vi "EnFlo_Hub.vi"() -> ()   [LabVIEW 2010]
uses:
  Anemometry Sub Vis/Controls/Launch_controls/Open_Calib.ctl
  Anemometry Sub Vis/Controls/Launch_controls/Open_Meas.ctl
  Anemometry Sub Vis/Controls/Launch_controls/Open_Enter_Temp.ctl
  Anemometry Sub Vis/Controls/Launch_controls/Multi_Run_Prog.ctl
  Anemometry Sub Vis/Controls/Launch_controls/EnFlo_arm.ctl
  Anemometry Sub Vis/Controls/Launch_controls/Fast_FID_Valve.ctl
  Anemometry Sub Vis/Controls/Launch_controls/Disp_Setup.ctl
  Anemometry Sub Vis/Controls/Launch_controls/EnFlo_Tun_Setup.ctl
  Anemometry Sub Vis/Controls/Launch_controls/User_Metadata.ctl
  Anemometry Sub Vis/Controls/Launch_controls/Trav_3D_move.ctl
  Anemometry Sub Vis/Controls/Launch_controls/Trav_Space.ctl
  Anemometry Sub Vis/Controls/Launch_controls/Tunnel_speed.ctl
  Anemometry Sub Vis/Controls/Launch_controls/Client_source_control.ctl
  Anemometry Sub Vis/Controls/Launch_controls/Hydrosonic_Manual.ctl
  Anemometry Sub Vis/Controls/Launch_controls/Preference_Panel.ctl
  Anemometry Sub Vis/Controls/Launch_controls/Hot_wire_Calculator.ctl
  Anemometry Sub Vis/Controls/Launch_controls/RW_X_Parker_Config.ctl
  Anemometry Sub Vis/Controls/Launch_controls/LDA_Alignment.ctl
  Anemometry Sub Vis/Controls/Launch_controls/Named_Serial_Comms.ctl
  Anemometry Sub Vis/Controls/Launch_controls/BSA_data_rates.ctl
  Anemometry Sub Vis/Controls/Launch_controls/Recompile_Code.ctl
  Anemometry Sub Vis/Controls/Launch_controls/Serial_Setup.ctl
  Anemometry Sub Vis/Controls/Launch_controls/Post_Process_icon.ctl
  Anemometry Sub Vis/Controls/Launch_controls/Edit_Ascii_file.ctl
  Anemometry Sub Vis/Controls/Launch_controls/Edit_Raw_DF.ctl
  Anemometry Sub Vis/Controls/Launch_controls/Results_file_plotter.ctl
  Anemometry Sub Vis/Controls/Launch_controls/Serial_Port_Names.ctl
  Anemometry Sub Vis/Controls/Launch_controls/Enter_LDA_Setup.ctl
  Anemometry Sub Vis/Controls/Launch_controls/Paul.ctl
  Anemometry Sub Vis/Controls/Launch_controls/Tom.ctl
  Anemometry Sub Vis/Controls/Launch_controls/Scani_Valve.ctl
  Anemometry Sub Vis/Controls/Launch_controls/Edit_sever_Channel.ctl
  Anemometry Sub Vis/Controls/Launch_controls/Day_file_plotter.ctl
  Anemometry Sub Vis/Controls/Launch_controls/Plot_Sever_Data.ctl
  Anemometry Sub Vis/Controls/Launch_controls/Adam_Table.ctl
  Anemometry Sub Vis/Controls/Launch_controls/Active_Channel_Control.ctl
  Anemometry Sub Vis/Controls/Post_Process.ctl
  Anemometry Sub Vis/Controls/Setup.ctl
  Anemometry Sub Vis/Controls/Preference_Mode.ctl
  Anemometry Sub Vis/Controls/User_Specific_mode.ctl
  Anemometry Sub Vis/Gen Trav/Trav_mode.ctl
  Anemometry Sub Vis/Calibration/Calib_mode.ctl
  Anemometry Sub Vis/Controls/App_Global.ctl
  Anemometry Sub Vis/Globals/Dynamic_call_global.ph.vi
  Anemometry Sub Vis/Globals/Preference_global.vi
  Anemometry Sub Vis/Globals/Constants_global.vi
  Anemometry Sub Vis/Globals/Meas_global.vi
  <vilib>/Platform/browser.llb/Open URL in Default Browser (string).vi
  Anemometry Sub Vis/Globals/Trav_pos_global.vi
  Anemometry Sub Vis/Acquisition/PWA/PWAtasksGLOBAL.vi
  Anemometry Sub Vis/Globals/Qnet_Globals.vi
  Anemometry Sub Vis/Utilities/Email_transfer_global.vi
panel:
  out "List of ADAM channels to view":string[](array[string])
  out "List of ADAM control channels":string[](array[string])
  out "Analogue Dev Name":string="Dev2"
  out "Numeric":i32
  out "Rig Name":string="EnFlo Tunnel"
  out "Meas setups folder":path=path "/System Folder/Preferences/LabVIEW (EnFlo specific)/Meas Setups"
  out "Dummy Measurement":bool
  out "Ready to take data?":T1
  out "Local Site Root":path=path "/Lacie_20/paulhayden/Qnet/qnet"
  in  "stop":bool
  in  "Tab Control":T2(tab)
  in  "Tunnel Speed Control":T3
  in  "Traverse Space":T4
  in  "Trav 3D Move":T5 caption="3D Traverse Move"
  in  "User Metadata":T6
  in  "Multi Run Prog":T7
  in  "Enter Temp_Press":T8
  in  "Measurement Prog":T9 caption="Measurement"
  in  "Calibration Prog":T10 caption="Calibration"
  in  "Scani Valve":T11
  in  "LDA Alignment":T12
  in  "Hydrosonic Control":T13
  in  "Fast FID Valve":T14
  in  "Source Control":T15
  in  "Gas Release Setup":T16
  in  "EnFlo Tunnel Setup":T17
  in  "Heater Setup":bool caption="Inlet heater File"
  in  "EnFlo Arm":T18
  in  "Rig_Control":cluster{"Ch Name":string, "Boolean":bool}[](array[cluster])
  in  "ADAM Channels Control":T19 caption="Change Active Channels"
  in  "ADAM Scan Table":T20 caption="Run ADAM Scan Table"
  in  "Edit Server Channel":T21
  in  "Plot Server Channels":T22 caption="Plot Server Data"
  in  "Day Files Plotter":T23 caption="Plot Data From File"
  out "Current Values":cluster{"Ch Name":string, "Numeric":dbl}[](array[cluster])
  in  "Results File Plotter":T24
  in  "Edit Raw Data Files":T25
  in  "Edit ASCII File":T26
  in  "Post Process Raw Data":T27
  in  "LDA Setup":T28
  in  "Port Names":T29
  in  "Serial Setup":T30
  in  "Software Update":T31
  in  "LDA Data Rate":T32
  in  "Named Serial Comms":T33
  in  "RW Trav Setup":T34
  in  "Hot Wire Calc":T35
  in  "Preference Panel":T36
  in  "Tom Lawton t.lawton@surrey.ac.uk":T37 caption="For hardware support"
  in  "Paul Hayden p.hayden@surrey.ac.uk":T38 caption="For software support"
  in  "Online Manual":bool
  out "VI Name":string
  out "Iterations":i32
  # "Or give us a call on Tel: 01483 689545"
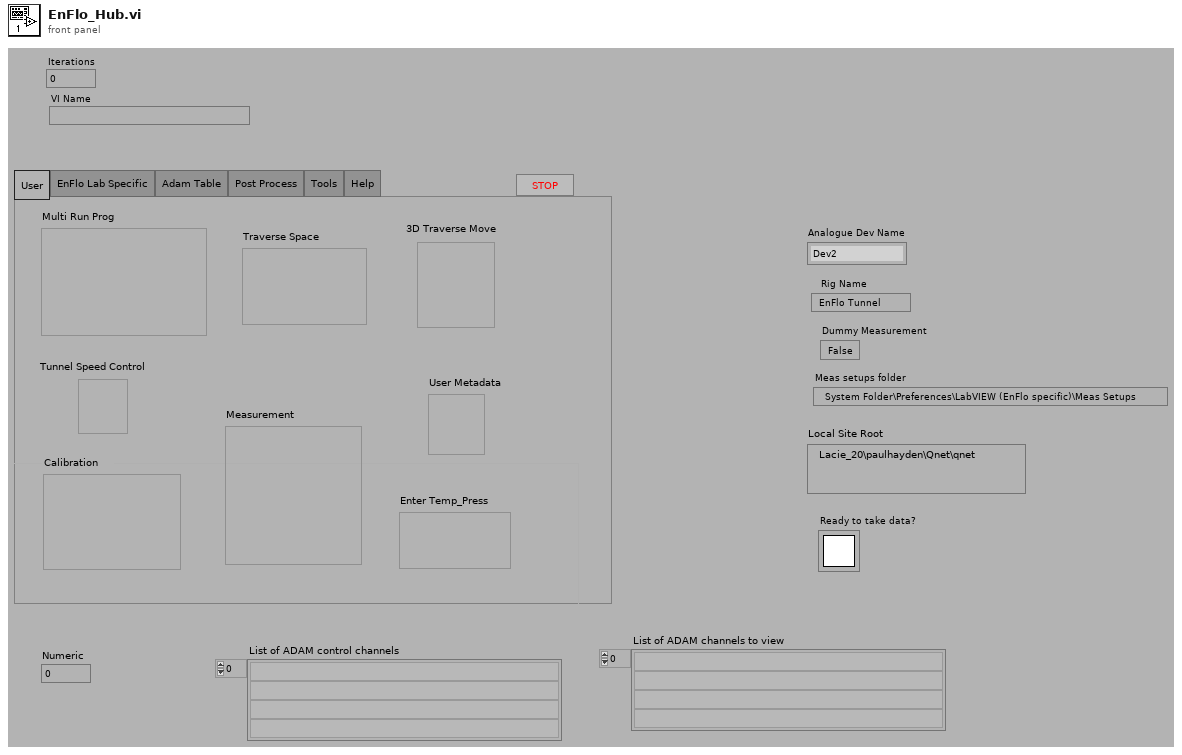
[diagram p1: front panel]
types:
  T1 = typedef "Rendezvous RefNum" = refnum<k1>
  T2 = enum32{"User", "EnFlo Lab Specific", "Adam Table", "Post Process", "Tools", "Help"}
  T3 = typedef "Tunnel_speed.ctl" = bool
  T4 = typedef "Trav_Space.ctl" = bool
  T5 = typedef "Trav_3D_move.ctl" = bool
  T6 = typedef "User_Metadata.ctl" = bool
  T7 = typedef "Multi_Run_Prog.ctl" = bool
  T8 = typedef "Open_Enter_Temp.ctl" = bool
  T9 = typedef "Open_Meas.ctl" = bool
  T10 = typedef "Open_Calib.ctl" = bool
  T11 = typedef "Scani_Valve.ctl" = bool
  T12 = typedef "LDA_Alignment.ctl" = bool
  T13 = typedef "Hydrosonic_Manual.ctl" = bool
  T14 = typedef "Fast_FID_Valve.ctl" = bool
  T15 = typedef "Client_source_control.ctl" = bool
  T16 = typedef "Disp_Setup.ctl" = bool
  T17 = typedef "EnFlo_Tun_Setup.ctl" = bool
  T18 = typedef "EnFlo_arm.ctl" = bool
  T19 = typedef "Active_Channel_Control.ctl" = bool
  T20 = typedef "Adam_Table.ctl" = bool
  T21 = typedef "Edit_sever_Channel.ctl" = bool
  T22 = typedef "Plot_Sever_Data.ctl" = bool
  T23 = typedef "Day_file_plotter.ctl" = bool
  T24 = typedef "Results_file_plotter.ctl" = bool
  T25 = typedef "Edit_Raw_DF.ctl" = bool
  T26 = typedef "Edit_Ascii_file.ctl" = bool
  T27 = typedef "Post_Process_icon.ctl" = bool
  T28 = typedef "Enter_LDA_Setup.ctl" = bool
  T29 = typedef "Serial_Port_Names.ctl" = bool
  T30 = typedef "Serial_Setup.ctl" = bool
  T31 = typedef "Recompile_Code.ctl" = bool
  T32 = typedef "BSA_data_rates.ctl" = bool
  T33 = typedef "Named_Serial_Comms.ctl" = bool
  T34 = typedef "RW_X_Parker_Config.ctl" = bool
  T35 = typedef "Hot_wire_Calculator.ctl" = bool
  T36 = typedef "Preference_Panel.ctl" = bool
  T37 = typedef "Tom.ctl" = bool
  T38 = typedef "Paul.ctl" = bool
  T39 = typedef "Post_Process.ctl" = enum16{"Take New Data", "Post Process Raw Data File"}
  T40 = typedef "Setup.ctl" = enum16{"Run Program", "Show Setup", "Save Current Setup", "Setup Front Panel"}
  T41 = enum16{"Get Channel Names", "Get Current Value", "Update Channel Value", "Update Channel Description"}
  T42 = typedef "Preference_Mode.ctl" = enum16{"Load Preferences from file", "Save Preferences to file", "Load, Edit then Save"}
  T43 = typedef "User_Specific_mode.ctl" = enum16{"Check VI only", "Run VI"}
  T44 = typedef "Trav_mode.ctl" = enum16{"Move traverse", "Read traverse position", "Teach Position"}
  T45 = enum16{"Load Command File", "Save Command File", "Check Multi Run Prog", "Check Multi Run Prog With Live Moves", "Run Multi Run Prog"}
  T46 = typedef "Calib_mode.ctl" = enum16{"Show Setup", "Take a New Calibration Point", "Refit Curve", "Setup Front Panel"}
  T47 = typedef "Tunnel_Coordinates.ctl" = enum16{"Work in Tunnel Coordinates", "Work in Model Coordinates"}
  T48 = typedef "App_Global.ctl" = enum16{"Read Global", "Write to Global", "Initialise Array"}
  T49 = typedef "App_Ref_Cluster.ctl" = cluster{"Server IP & Port No":string, "Application reference":refnum<vi>}
  T50 = typedef "Ch_description_ADAM.ctl" = cluster{"Ch Name":string, "Type":T51, "Function":T52, "Ch State":T53, "Calibration type":T54, "A":dbl, "B":dbl, "C":dbl, "D":dbl, "Comments":string, "Address":T55, "String":string, "Duty":u16}
  T51 = typedef "Module_type_ADAM.ctl" = enum16{"4011", "4012", "4013", "4014", "4016", "4017", "4018", "4021", "4050", "4052", "4053", "4060", "4080", "5000", "5017", "5018", "5024", "5051", "5056", "5060", "6060", "Tracker", "WEST", "GILL", "JEM", "VICI", "Vaisala", "DRUCK", "Run VI Named:", "IR2100", "PPT", "Comparator", "VIRTUAL", "Hold Value", "Read A", "Read Ch", "Coded", "Client Info", "Web Client", "X10", "Test"}
  T52 = typedef "Function_ADAM.ctl" = enum16{"Analogue Input", "Digital Input", "Event counter", "Event rate", "Analogue Output", "Digital Output", "Relay Output"}
  T53 = typedef "Channel_State.ctl" = enum16{"On", "Off", "Always On", "Always Off"}
  T54 = typedef "Calib_type_ADAM.ctl" = enum16{"Raw", "Bx + A", "Cx^2 + Bx + A", "Dx^3 + Cx^2 + Bx + A", "In Band", "Hi-Tec Q", "Hi-Tec M_dot", "Text"}
  T55 = typedef "Address.ctl" = cluster{"Main":i32, "Ch.":i32, "Sub":i32, "Port Name":string}
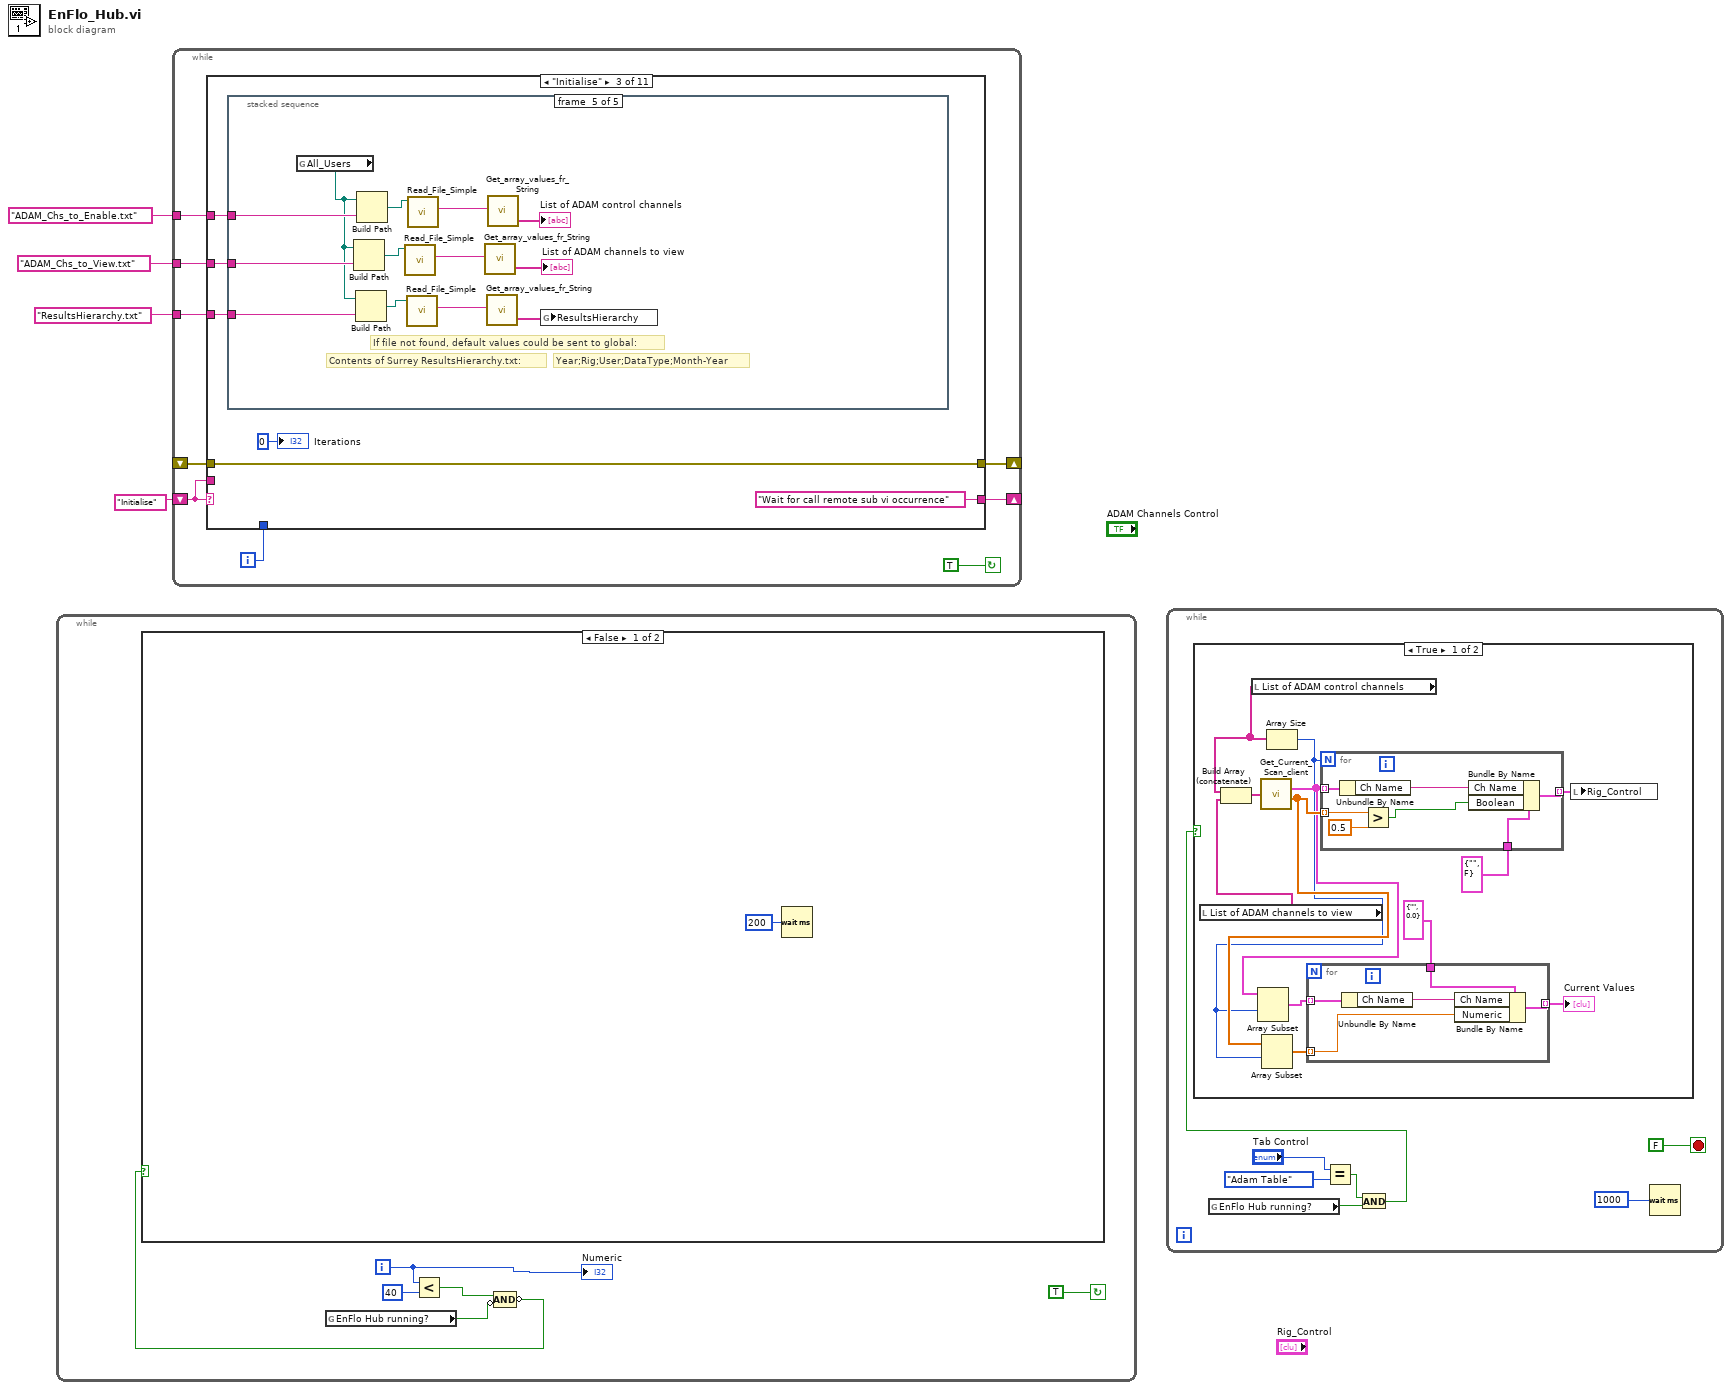
[diagram p0: block diagram]
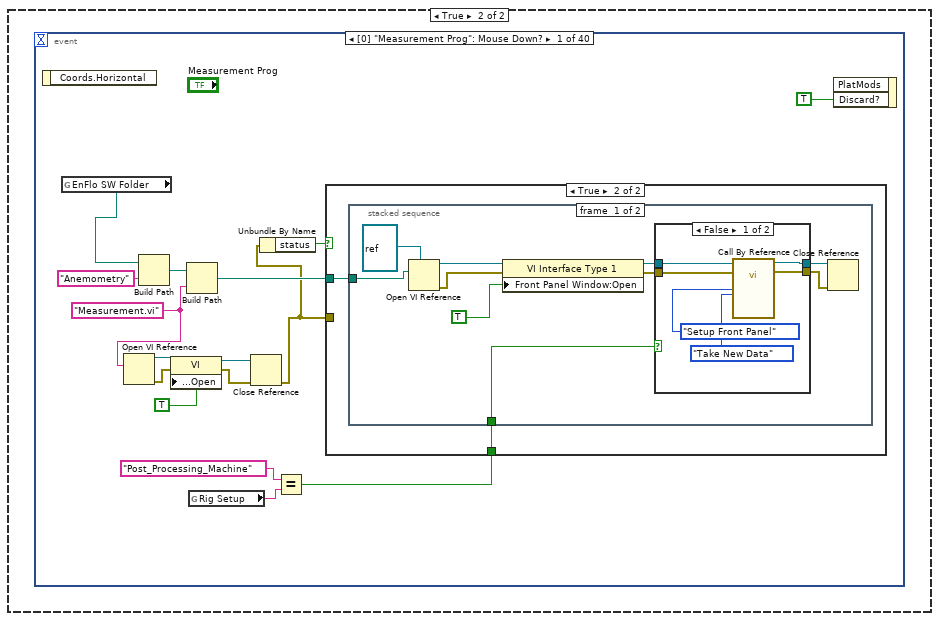
[diagram p3: hidden frame]
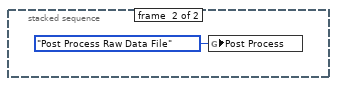
[diagram p6: hidden frame]
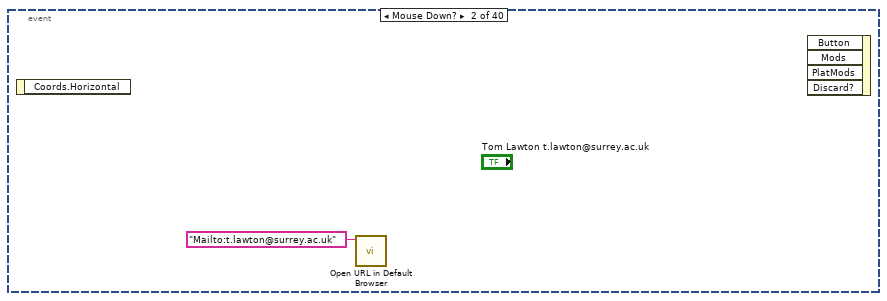
[diagram p7: hidden frame]
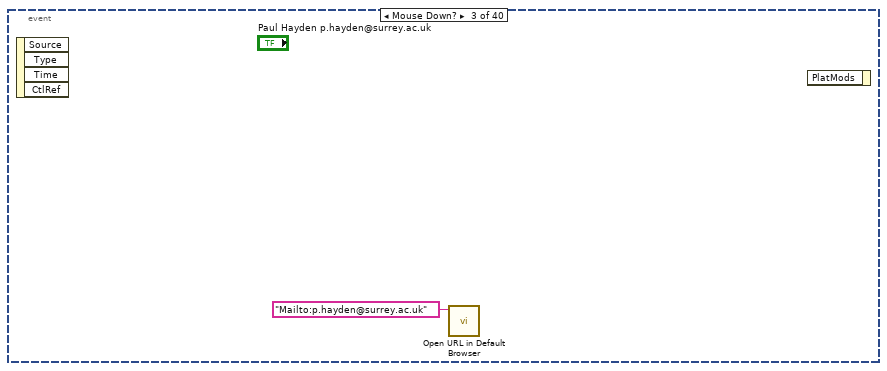
[diagram p8: hidden frame]
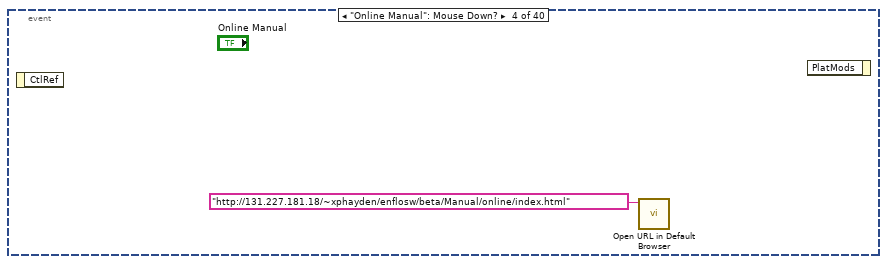
[diagram p9: hidden frame]
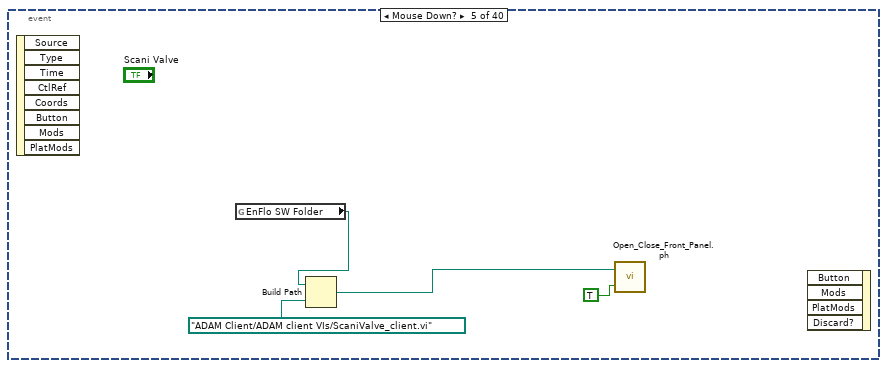
[diagram p10: hidden frame]
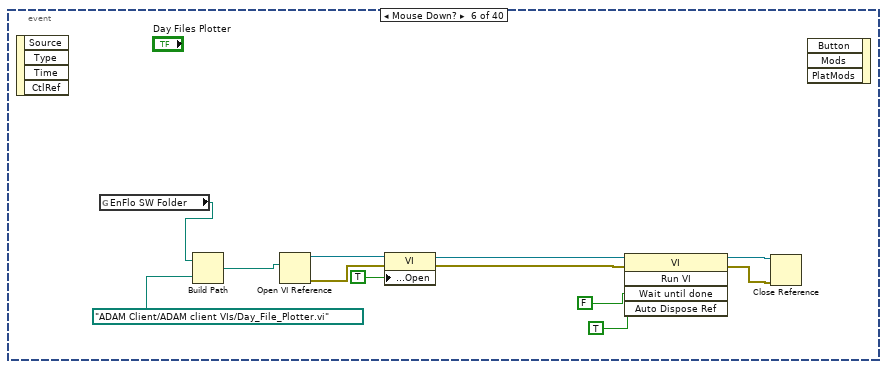
[diagram p11: hidden frame]
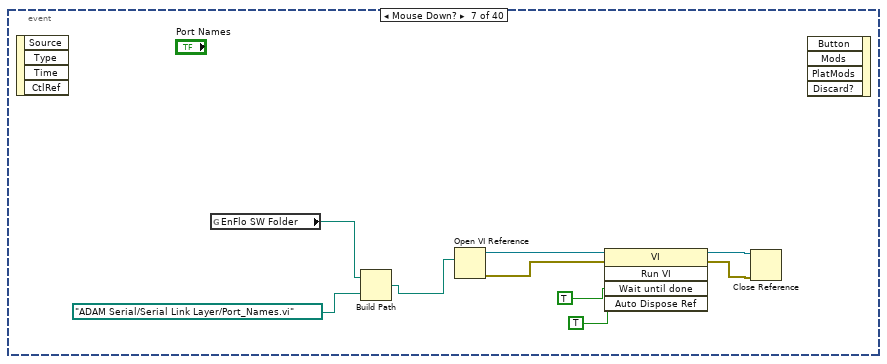
[diagram p12: hidden frame]
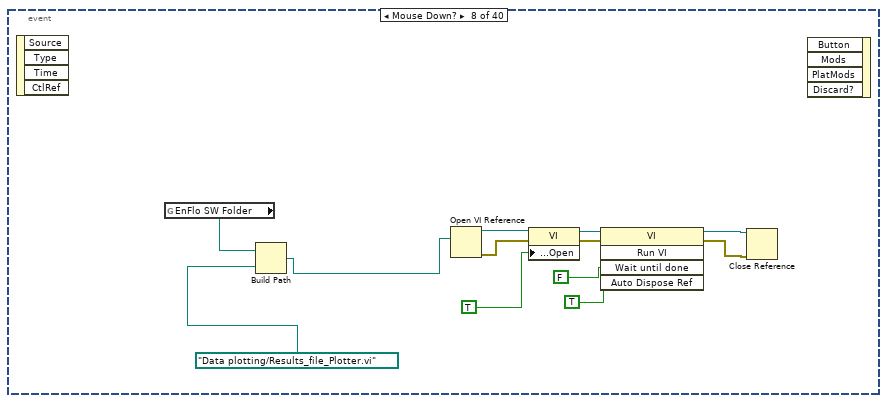
[diagram p13: hidden frame]
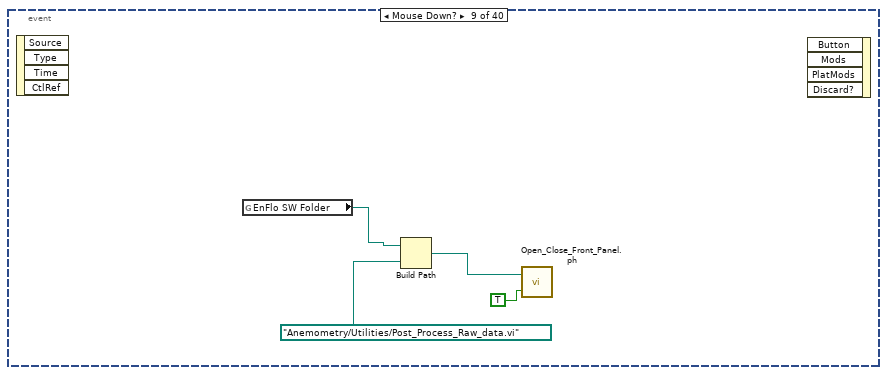
[diagram p14: hidden frame]
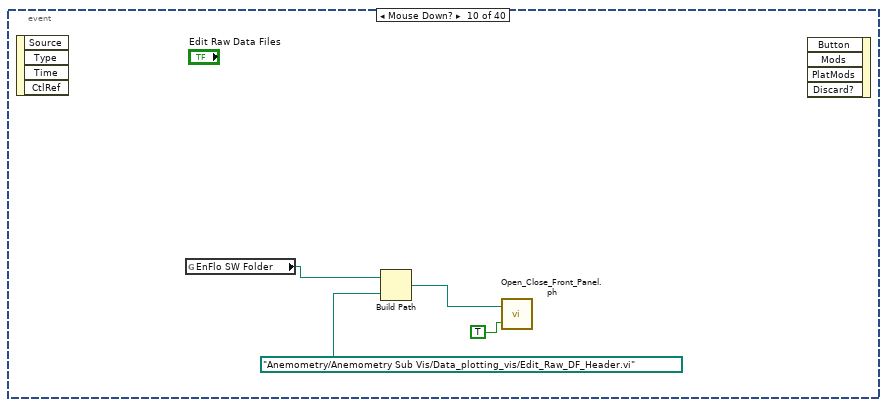
[diagram p15: hidden frame]
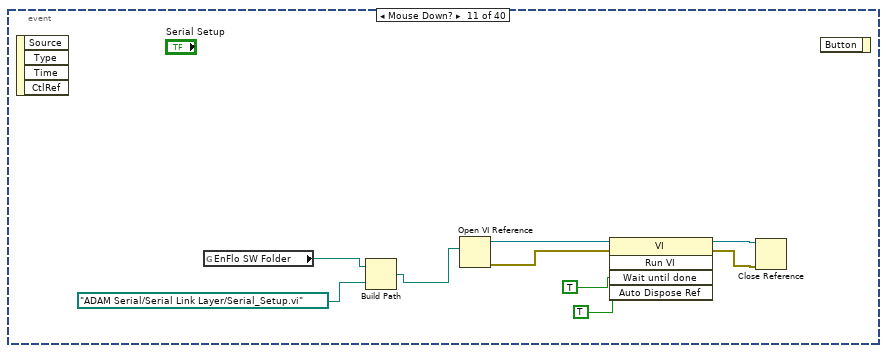
[diagram p16: hidden frame]
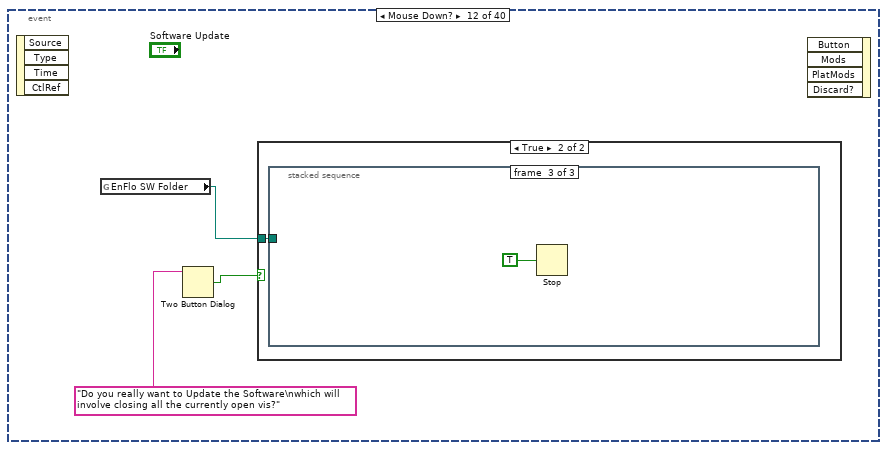
[diagram p17: hidden frame]
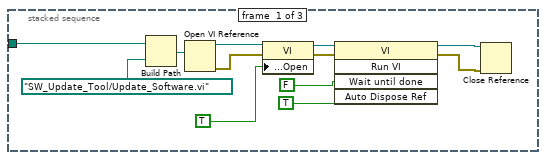
[diagram p19: hidden frame]
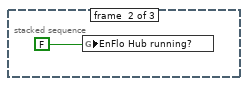
[diagram p20: hidden frame]
diagram:
  n1 = while {
    i -> [w9]
    stop <- TRUE continue-if-true
    n2 = global read "Dynamic_call_global.ph.vi" "EnFlo Hub running?"() -> (w7:bool)
    n3 = Less?(x=w9, y=40) -> (x < y?=w6:bool)
    n4 = Compound Arithmetic op=AND(w6, invert w7) -> (invert w5:bool)
    n5 = case shown="False" w5 {
      frame False {
        n6 = Wait (ms)(milliseconds to wait=u32 200) -> ()  [unwired: 1 out]
      }
      frame True {
        n7 = event shown="[0] \"Measurement Prog\": Mouse Down?" {
          selector: _ -> [_ _ _ _ _ _ _ _ _ _ _ _ _ _ _ _ _ _ _ _ _ _ _ _ _ _ _ _ _ _ _ _ _ _ _ _ _ _ _ _]
          dyn-events: _ -> [_ _ _ _ _ _ _ _ _ _ _ _ _ _ _ _ _ _ _ _ _ _ _ _ _ _ _ _ _ _ _ _ _ _ _ _ _ _ _ _]
          timeout: _ -> [_ _ _ _ _ _ _ _ _ _ _ _ _ _ _ _ _ _ _ _ _ _ _ _ _ _ _ _ _ _ _ _ _ _ _ _ _ _ _ _]
          event Mouse Down? {
            w20 = "Measurement.vi" ("name or relative path")
            n8 = event-data() -> ()  [unwired: 2 out]
            n9 = global read "Constants_global.vi" "EnFlo SW Folder"() -> (w23:path)
            n10 = Open VI Reference(vi path=w20) -> (vi reference=w19:refnum<vi>, error out=w18:errorcluster)  [unwired: 1 in, 4 out]
            n11 = Build Path(base path=w23, name or relative path="Anemometry") -> (appended path=w26:path)
            n12 = property class="VI"(reference=w19, error in=w18, "Front Panel Window:Open"=TRUE) -> (reference out=w16:refnum<vi>, error out=w17:errorcluster)
            n13 = Build Path(base path=w26, name or relative path=w20) -> (appended path=w24:path)
            n14 = global read "Preference_global.vi" "Rig Setup"() -> (w14:string)
            n15 = Close Reference(reference=w16, error in (no error)=w17) -> (error out=w15:errorcluster)
            n16 = Unbundle By Name(w15) -> ("status"=w25:bool)
            n17 = Equal?(x="Post_Processing_Machine" ("Rig Setup"), y=w14) -> (x = y?=w12:bool)
            n18 = case shown="True" w25 {
              tunnel: w24 -> [_ w29]
              tunnel: w15 -> [_ _]
              tunnel: w12 -> [_ w28]
              frame False {
              }
              frame True {
                n19 = stacked-sequence {
                  tunnel: w29 -> [w39 _]
                  tunnel: w28 -> [w30 _]
                  frame #0 {
                    n20 = Open VI Reference(type specifier VI Refnum (for type only)=refnum<vi> refnum, vi path=w39) -> (vi reference=w37:refnum<vi>, error out=w36:errorcluster)  [unwired: 1 in, 3 out]
                    n21 = property class="VI Interface Type 1"(reference=w37, error in=w36, "Front Panel Window:Open"=TRUE) -> (reference out=w32:refnum<vi>, error out=w31:errorcluster)
                    n22 = case shown="False" w30 {
                      tunnel: [w45 w47] -> w35
                      tunnel: [w44 w46] -> w34
                      tunnel: w32 -> [w43 w47]
                      tunnel: w31 -> [w42 w46]
                      frame False {
                        n23 = call-by-ref "?"(reference=w43, error in=w42, "setup"=Setup."Setup Front Panel", "Post Process"=Post_Process."Take New Data") -> (reference out=w45:refnum<vi>, error out=w44:errorcluster)  [unwired: 16 in, 2 out]
                      }
                      frame True {
                      }
                    }
                    n24 = Close Reference(reference=w35, error in (no error)=w34) -> ()  [unwired: 1 out]
                  }
                  frame #1 {
                    n25 = global write "Meas_global.vi" "Post Process"(Post_Process."Post Process Raw Data File" ("Post Process")) -> ()
                  }
                }
              }
            }
            n26 = event-data("Discard?"=TRUE) -> ()  [unwired: 1 in, 2 out]
          }
          event Mouse Down? {
            n27 = event-data() -> ()  [unwired: 2 out]
            n28 = call-poly <vilib>:"Open URL in Default Browser.vi"("URL"="Mailto:t.lawton@surrey.ac.uk") -> ()  [unwired: 1 in, 6 out]
            n29 = event-data() -> ()  [unwired: 1 in, 5 out]
          }
          event Mouse Down? {
            n30 = event-data() -> ()  [unwired: 5 out]
            n31 = call-poly <vilib>:"Open URL in Default Browser.vi"("URL"="Mailto:p.hayden@surrey.ac.uk") -> ()  [unwired: 1 in, 6 out]
            n32 = event-data() -> ()  [unwired: 1 in, 2 out]
          }
          event "Online Manual": Mouse Down? {
            n33 = event-data() -> ()  [unwired: 2 out]
            n34 = call-poly <vilib>:"Open URL in Default Browser.vi"("URL"="http://131.227.181.18/~xphayden/enflosw/beta/Manual/online/index.html") -> ()  [unwired: 1 in, 6 out]
            n35 = event-data() -> ()  [unwired: 1 in, 2 out]
          }
          event Mouse Down? {
            n36 = event-data() -> ()  [unwired: 9 out]
            n37 = global read "Constants_global.vi" "EnFlo SW Folder"() -> (w52:path)
            n38 = Build Path(base path=w52, name or relative path=path "ADAM Client/ADAM client VIs/ScaniValve_client.vi") -> (appended path=w55:path)
            n39 = call "Open_Close_Front_Panel.ph.vi"("Front Panel Window:Open"=TRUE, "VI path"=w55) -> ()  [unwired: 2 out]
            n40 = event-data() -> ()  [unwired: 1 in, 5 out]
          }
          event Mouse Down? {
            n41 = event-data() -> ()  [unwired: 5 out]
            n42 = global read "Constants_global.vi" "EnFlo SW Folder"() -> (w56:path)
            n43 = Build Path(base path=w56, name or relative path=path "ADAM Client/ADAM client VIs/Day_File_Plotter.vi") -> (appended path=w62:path)
            n44 = Open VI Reference(vi path=w62) -> (vi reference=w63:refnum<vi>, error out=w65:errorcluster)  [unwired: 2 in, 3 out]
            n45 = property class="VI"(reference=w63, error in=w65, "Front Panel Window:Open"=TRUE) -> (reference out=w67:refnum<vi>, error out=w66:errorcluster)
            n46 = invoke class="VI" method="Run VI"(reference=w67, error in=w66, "Wait until done"=FALSE, "Auto Dispose Ref"=TRUE) -> (reference out=w58:refnum<vi>, error out=w59:errorcluster)  [unwired: 1 in, 3 out]
            n47 = Close Reference(reference=w58, error in (no error)=w59) -> ()  [unwired: 1 out]
            n48 = event-data() -> ()  [unwired: 1 in, 4 out]
          }
          event Mouse Down? {
            n49 = event-data() -> ()  [unwired: 5 out]
            n50 = global read "Constants_global.vi" "EnFlo SW Folder"() -> (w68:path)
            n51 = Build Path(base path=w68, name or relative path=path "ADAM Serial/Serial Link Layer/Port_Names.vi") -> (appended path=w70:path)
            n52 = Open VI Reference(vi path=w70) -> (vi reference=w75:refnum<vi>, error out=w76:errorcluster)  [unwired: 1 in, 4 out]
            n53 = invoke class="VI" method="Run VI"(reference=w75, error in=w76, "Wait until done"=TRUE, "Auto Dispose Ref"=TRUE) -> (reference out=w71:refnum<vi>, error out=w72:errorcluster)  [unwired: 1 in, 3 out]
            n54 = Close Reference(reference=w71, error in (no error)=w72) -> ()  [unwired: 1 out]
            n55 = event-data() -> ()  [unwired: 1 in, 5 out]
          }
          event Mouse Down? {
            n56 = event-data() -> ()  [unwired: 5 out]
            n57 = global read "Constants_global.vi" "EnFlo SW Folder"() -> (w77:path)
            n58 = Build Path(base path=w77, name or relative path=path "Data plotting/Results_file_Plotter.vi") -> (appended path=w80:path)
            n59 = Open VI Reference(vi path=w80) -> (vi reference=w82:refnum<vi>, error out=w79:errorcluster)  [unwired: 1 in, 4 out]
            n60 = property class="VI"(reference=w82, error in=w79, "Front Panel Window:Open"=TRUE) -> (reference out=w83:refnum<vi>, error out=w84:errorcluster)
            n61 = invoke class="VI" method="Run VI"(reference=w83, error in=w84, "Wait until done"=FALSE, "Auto Dispose Ref"=TRUE) -> (reference out=w85:refnum<vi>, error out=w86:errorcluster)  [unwired: 1 in, 3 out]
            n62 = Close Reference(reference=w85, error in (no error)=w86) -> ()  [unwired: 1 out]
            n63 = event-data() -> ()  [unwired: 1 in, 5 out]
          }
          event Mouse Down? {
            n64 = event-data() -> ()  [unwired: 5 out]
            n65 = global read "Constants_global.vi" "EnFlo SW Folder"() -> (w89:path)
            n66 = Build Path(base path=w89, name or relative path=path "Anemometry/Utilities/Post_Process_Raw_data.vi") -> (appended path=w91:path)
            n67 = call "Open_Close_Front_Panel.ph.vi"("Front Panel Window:Open"=TRUE, "VI path"=w91) -> ()  [unwired: 2 out]
            n68 = event-data() -> ()  [unwired: 1 in, 5 out]
          }
          event Mouse Down? {
            n69 = event-data() -> ()  [unwired: 5 out]
            n70 = global read "Constants_global.vi" "EnFlo SW Folder"() -> (w93:path)
            n71 = Build Path(base path=w93, name or relative path=path "Anemometry/Anemometry Sub Vis/Data_plotting_vis/Edit_Raw_DF_Header.vi") -> (appended path=w95:path)
            n72 = call "Open_Close_Front_Panel.ph.vi"("Front Panel Window:Open"=TRUE, "VI path"=w95) -> ()  [unwired: 2 out]
            n73 = event-data() -> ()  [unwired: 1 in, 5 out]
          }
          event Mouse Down? {
            n74 = event-data() -> ()  [unwired: 5 out]
            n75 = global read "Constants_global.vi" "EnFlo SW Folder"() -> (w97:path)
            n76 = Build Path(base path=w97, name or relative path=path "ADAM Serial/Serial Link Layer/Serial_Setup.vi") -> (appended path=w99:path)
            n77 = Open VI Reference(vi path=w99) -> (vi reference=w104:refnum<vi>, error out=w105:errorcluster)  [unwired: 1 in, 4 out]
            n78 = invoke class="VI" method="Run VI"(reference=w104, error in=w105, "Wait until done"=TRUE, "Auto Dispose Ref"=TRUE) -> (reference out=w100:refnum<vi>, error out=w101:errorcluster)  [unwired: 1 in, 3 out]
            n79 = Close Reference(reference=w100, error in (no error)=w101) -> ()  [unwired: 1 out]
            n80 = event-data() -> ()  [unwired: 1 in, 2 out]
          }
          event Mouse Down? {
            n81 = event-data() -> ()  [unwired: 5 out]
            n82 = global read "Constants_global.vi" "EnFlo SW Folder"() -> (w106:path)
            n83 = Two Button Dialog(message="Do you really want to Update the Software\nwhich will involve closing all the currently open vis?") -> (T button?=w108:bool)  [unwired: 2 out]
            n84 = case shown="True" w108 {
              tunnel: w106 -> [_ w109]
              frame False {
              }
              frame True {
                n85 = stacked-sequence {
                  tunnel: w109 -> [w121 _ _]
                  frame #0 {
                    n86 = Build Path(base path=w121, name or relative path=path "SW_Update_Tool/Update_Software.vi") -> (appended path=w119:path)
                    n87 = Open VI Reference(vi path=w119) -> (vi reference=w117:refnum<vi>, error out=w120:errorcluster)  [unwired: 1 in, 4 out]
                    n88 = property class="VI"(reference=w117, error in=w120, "Front Panel Window:Open"=TRUE) -> (reference out=w116:refnum<vi>, error out=w115:errorcluster)
                    n89 = invoke class="VI" method="Run VI"(reference=w116, error in=w115, "Wait until done"=FALSE, "Auto Dispose Ref"=TRUE) -> (reference out=w114:refnum<vi>, error out=w113:errorcluster)  [unwired: 1 in, 3 out]
                    n90 = Close Reference(reference=w114, error in (no error)=w113) -> ()  [unwired: 1 out]
                  }
                  frame #1 {
                    n91 = global write "Dynamic_call_global.ph.vi" "EnFlo Hub running?"(FALSE ("EnFlo Hub running?")) -> ()
                  }
                  frame #2 {
                    n92 = Stop(stop? (T)=TRUE) -> ()
                  }
                }
              }
            }
            n93 = event-data() -> ()  [unwired: 1 in, 5 out]
          }
          event Mouse Down? {
            n94 = event-data() -> ()  [unwired: 5 out]
            n95 = global read "Constants_global.vi" "EnFlo SW Folder"() -> (w125:path)
            n96 = Build Path(base path=w125, name or relative path=path "ADAM Serial/Serial Link Layer/Named_Serial_Comms.vi") -> (appended path=w127:path)
            n97 = call "Open_Close_Front_Panel.ph.vi"("Front Panel Window:Open"=TRUE, "VI path"=w127) -> ()  [unwired: 2 out]
            n98 = event-data() -> ()  [unwired: 1 in, 5 out]
          }
          event Mouse Down? {
            n99 = event-data() -> ()  [unwired: 5 out]
            n100 = global read "Constants_global.vi" "EnFlo SW Folder"() -> (w128:path)
            n101 = Build Path(base path=w128, name or relative path=path "Anemometry/Anemometry Sub Vis/LDA/LDA_data_rate.vi") -> (appended path=w130:path)
            n102 = call "Open_Close_Front_Panel.ph.vi"("Front Panel Window:Open"=TRUE, "VI path"=w130) -> ()  [unwired: 2 out]
            n103 = event-data() -> ()  [unwired: 1 in, 2 out]
          }
          event Mouse Down? {
            n104 = event-data() -> ()  [unwired: 5 out]
            n105 = global read "Constants_global.vi" "EnFlo SW Folder"() -> (w142:path)
            n106 = Build Path(base path=w142, name or relative path=path "ADAM Client/ADAM client VIs/Control_Channel_Status.vi") -> (appended path=w132:path)
            n107 = Open VI Reference(vi path=w132) -> (vi reference=w135:refnum<vi>, error out=w133:errorcluster)  [unwired: 1 in, 4 out]
            n108 = property class="VI"(reference=w135, error in=w133, "Front Panel Window:Open"=TRUE) -> (reference out=w136:refnum<vi>, error out=w137:errorcluster)
            n109 = invoke class="VI" method="Run VI"(reference=w136, error in=w137, "Wait until done"=FALSE, "Auto Dispose Ref"=TRUE) -> (reference out=w138:refnum<vi>, error out=w139:errorcluster)  [unwired: 1 in, 3 out]
            n110 = Close Reference(reference=w138, error in (no error)=w139) -> ()  [unwired: 1 out]
            n111 = event-data() -> ()  [unwired: 1 in, 2 out]
          }
          event Mouse Down? {
            n112 = event-data() -> ()  [unwired: 5 out]
            n113 = global read "Constants_global.vi" "EnFlo SW Folder"() -> (w144:path)
            n114 = Build Path(base path=w144, name or relative path=path "Anemometry/Utilities/LDA_Beam_Alignment.vi") -> (appended path=w146:path)
            n115 = call "Open_Close_Front_Panel.ph.vi"("Front Panel Window:Open"=TRUE, "VI path"=w146) -> ()  [unwired: 2 out]
            n116 = event-data() -> ()  [unwired: 1 in, 5 out]
          }
          event Mouse Down? {
            w149 = FALSE  # Wait until done
            n117 = event-data() -> ()  [unwired: 5 out]
            n118 = call "Run_Enter_Temp.vi"("Wait until done"=w149) -> ()  [unwired: 1 out]
            n119 = event-data("Discard?"=TRUE) -> ()  [unwired: 1 in, 4 out]
          }
          event Mouse Down? {
            n120 = event-data() -> ()  [unwired: 5 out]
            n121 = global read "Constants_global.vi" "EnFlo SW Folder"() -> (w150:path)
            n122 = Build Path(base path=w150, name or relative path=path "Anemometry/Utilities/Edit_ASCI_file.vi") -> (appended path=w153:path)
            n123 = call "Open_Close_Front_Panel.ph.vi"("Front Panel Window:Open"=TRUE, "VI path"=w153) -> ()  [unwired: 2 out]
            n124 = event-data() -> ()  [unwired: 1 in, 5 out]
          }
          event "Heater Setup": Mouse Down? {
            n125 = event-data() -> ()  [unwired: 5 out]
            n126 = global read "Constants_global.vi" "EnFlo SW Folder"() -> (w154:path)
            n127 = Build Path(base path=w154, name or relative path=path "Anemometry/Utilities/Create_Heater_Setpoints_File.vi") -> (appended path=w157:path)
            n128 = call "Open_Close_Front_Panel.ph.vi"("Front Panel Window:Open"=TRUE, "VI path"=w157) -> ()  [unwired: 2 out]
            n129 = event-data() -> ()  [unwired: 1 in, 5 out]
          }
          event Mouse Down? {
            n130 = event-data() -> ()  [unwired: 5 out]
            n131 = global read "Constants_global.vi" "EnFlo SW Folder"() -> (w158:path)
            n132 = Build Path(base path=w158, name or relative path=path "ADAM Client/Sub VIs/Gas_Release_Control.vi") -> (appended path=w161:path)
            n133 = call "Open_Close_Front_Panel.ph.vi"("Front Panel Window:Open"=TRUE, "VI path"=w161) -> ()  [unwired: 2 out]
            n134 = event-data() -> ()  [unwired: 1 in, 5 out]
          }
          event Mouse Down? {
            n135 = event-data() -> ()  [unwired: 5 out]
            n136 = global read "Constants_global.vi" "EnFlo SW Folder"() -> (w162:path)
            n137 = Build Path(base path=w162, name or relative path=path "ADAM Client/ADAM client VIs/Edit_Server_Channel.vi") -> (appended path=w172:path)
            n138 = Open VI Reference(type specifier VI Refnum (for type only)=refnum<vi> refnum, vi path=w172) -> (vi reference=w165:refnum<vi>, error out=w166:errorcluster)  [unwired: 1 in, 3 out]
            n139 = property class="VI Interface Type 2"(reference=w165, error in=w166, "Front Panel Window:Open"=TRUE) -> (reference out=w168:refnum<vi>, error out=w169:errorcluster)
            n140 = call-by-ref "?"(reference=w168, error in=w169, "Mode"=T41."Get Channel Names") -> (reference out=w170:refnum<vi>, error out=w171:errorcluster)  [unwired: 5 in]
            n141 = Close Reference(reference=w170, error in (no error)=w171) -> ()  [unwired: 1 out]
            n142 = event-data() -> ()  [unwired: 1 in, 5 out]
          }
          event Mouse Down? {
            n143 = event-data() -> ()  [unwired: 5 out]
            n144 = global read "Constants_global.vi" "EnFlo SW Folder"() -> (w174:path)
            n145 = Build Path(base path=w174, name or relative path=path "ADAM Client/ADAM client VIs/Set_Tunnel_Speed.vi") -> (appended path=w177:path)
            n146 = call "Open_Close_Front_Panel.ph.vi"("Front Panel Window:Open"=TRUE, "VI path"=w177) -> ()  [unwired: 2 out]
            n147 = event-data() -> ()  [unwired: 1 in, 5 out]
          }
          event Mouse Down? {
            n148 = event-data() -> ()  [unwired: 5 out]
            n149 = global read "Constants_global.vi" "EnFlo SW Folder"() -> (w178:path)
            n150 = Build Path(base path=w178, name or relative path=path "ADAM Client/ADAM client VIs/Plot_Server_Data.vi") -> (appended path=w181:path)
            n151 = Open VI Reference(vi path=w181) -> (vi reference=w183:refnum<vi>, error out=w180:errorcluster)  [unwired: 1 in, 4 out]
            n152 = property class="VI"(reference=w183, error in=w180, "Front Panel Window:Open"=TRUE) -> (reference out=w184:refnum<vi>, error out=w185:errorcluster)
            n153 = invoke class="VI" method="Run VI"(reference=w184, error in=w185, "Wait until done"=FALSE, "Auto Dispose Ref"=TRUE) -> (reference out=w186:refnum<vi>, error out=w187:errorcluster)  [unwired: 1 in, 3 out]
            n154 = Close Reference(reference=w186, error in (no error)=w187) -> ()  [unwired: 1 out]
            n155 = event-data() -> ()  [unwired: 1 in, 5 out]
          }
          event Mouse Down? {
            n156 = event-data() -> ()  [unwired: 5 out]
            n157 = Two Button Dialog(message="Are you sure that you want to Run the ADAM Scan table on this machine?", 1:"Run" ("F button name (\"Cancel\")"), 2:"Cancel" ("T button name (\"OK\")")) -> (T button?=w191:bool)
            n158 = case shown="False" w191 {
              frame False {
                n159 = global read "Constants_global.vi" "EnFlo SW Folder"() -> (w194:path)
                n160 = Build Path(base path=w194, name or relative path=path "ADAM Server/ADAM_scan_table.vi") -> (appended path=w197:path)
                n161 = Open VI Reference(vi path=w197) -> (vi reference=w199:refnum<vi>, error out=w196:errorcluster)  [unwired: 1 in, 4 out]
                n162 = property class="VI"(reference=w199, error in=w196, "Front Panel Window:Open"=TRUE) -> (reference out=w200:refnum<vi>, error out=w201:errorcluster)
                n163 = invoke class="VI" method="Run VI"(reference=w200, error in=w201, "Wait until done"=FALSE, "Auto Dispose Ref"=TRUE) -> (reference out=w202:refnum<vi>, error out=w203:errorcluster)  [unwired: 1 in, 3 out]
                n164 = Close Reference(reference=w202, error in (no error)=w203) -> ()  [unwired: 1 out]
              }
              frame True {
              }
            }
            n165 = event-data() -> ()  [unwired: 1 in, 2 out]
          }
          event Mouse Down? {
            n166 = event-data() -> ()  [unwired: 5 out]
            n167 = global read "Constants_global.vi" "EnFlo SW Folder"() -> (w208:path)
            n168 = Build Path(base path=w208, name or relative path=path "ADAM Serial/Instrument drivers/Traverses/~subVIs/Read_Write_Trav_Config.vi") -> (appended path=w209:path)
            n169 = Build Path(base path=w208, name or relative path=path "ADAM Serial/Instrument drivers/Traverses/~subVIs/DriveConfigGlobal.vi") -> (appended path=w210:path)
            n170 = flat-sequence {
              tunnel: w210 -> [w211]
              tunnel: w209 -> [w213]
              frame #0 {
                n171 = call "Open_Close_Front_Panel.ph.vi"("Front Panel Window:Open"=TRUE, "VI path"=w211) -> ()  [unwired: 2 out]
              }
              frame #1 {
                n172 = call "Open_Close_Front_Panel.ph.vi"("Front Panel Window:Open"=TRUE, "VI path"=w213) -> ()  [unwired: 2 out]
              }
            }
            n173 = event-data() -> ()  [unwired: 1 in, 5 out]
          }
          event Mouse Down? {
            n174 = event-data() -> ()  [unwired: 5 out]
            n175 = global read "Constants_global.vi" "EnFlo SW Folder"() -> (w215:path)
            n176 = Build Path(base path=w215, name or relative path=path "Anemometry/Utilities/Hot_wire_Calculator.vi") -> (appended path=w218:path)
            n177 = call "Open_Close_Front_Panel.ph.vi"("Front Panel Window:Open"=TRUE, "VI path"=w218) -> ()  [unwired: 2 out]
            n178 = event-data() -> ()  [unwired: 1 in, 5 out]
          }
          event Mouse Down? {
            n179 = event-data() -> ()  [unwired: 5 out]
            n180 = global read "Constants_global.vi" "EnFlo SW Folder"() -> (w219:path)
            n181 = Build Path(base path=w219, name or relative path=path "Anemometry/Utilities/Hydrosonic_Manual.vi") -> (appended path=w222:path)
            n182 = call "Open_Close_Front_Panel.ph.vi"("Front Panel Window:Open"=TRUE, "VI path"=w222) -> ()  [unwired: 2 out]
            n183 = event-data() -> ()  [unwired: 1 in, 5 out]
          }
          event Mouse Down? {
            n184 = event-data() -> ()  [unwired: 5 out]
            n185 = global read "Constants_global.vi" "EnFlo SW Folder"() -> (w223:path)
            n186 = Build Path(base path=w223, name or relative path=path "ADAM Client/ADAM client VIs/Fast_FID_Valve_Control.vi") -> (appended path=w226:path)
            n187 = call "Open_Close_Front_Panel.ph.vi"("Front Panel Window:Open"=TRUE, "VI path"=w226) -> ()  [unwired: 2 out]
            n188 = event-data() -> ()  [unwired: 1 in, 5 out]
          }
          event Mouse Down? {
            n189 = event-data() -> ()  [unwired: 5 out]
            n190 = global read "Constants_global.vi" "EnFlo SW Folder"() -> (w227:path)
            n191 = Build Path(base path=w227, name or relative path=path "Anemometry/Utilities/Preference_Panel.vi") -> (appended path=w236:path)
            n192 = Open VI Reference(type specifier VI Refnum (for type only)=refnum<vi> refnum, vi path=w236) -> (vi reference=w229:refnum<vi>, error out=w230:errorcluster)  [unwired: 1 in, 3 out]
            n193 = property class="VI Interface Type 3"(reference=w229, error in=w230, "Front Panel Window:Open"=TRUE) -> (reference out=w232:refnum<vi>, error out=w233:errorcluster)
            n194 = call-by-ref "?"(reference=w232, error in=w233, "Mode"=Preference_Mode."Load, Edit then Save") -> (reference out=w234:refnum<vi>, error out=w235:errorcluster)
            n195 = Close Reference(reference=w234, error in (no error)=w235) -> ()  [unwired: 1 out]
            n196 = event-data("Discard?"=TRUE) -> ()  [unwired: 1 in, 4 out]
          }
          event Mouse Down? {
            n197 = event-data() -> ()  [unwired: 5 out]
            n198 = global read "Constants_global.vi" "EnFlo SW Folder"() -> (w243:path)
            n199 = Build Path(base path=w243, name or relative path=path "ADAM Client/Sub VIs/Gas_Setup.vi") -> (appended path=w250:path)
            n200 = Open VI Reference(type specifier VI Refnum (for type only)=refnum<vi> refnum, vi path=w250) -> (vi reference=w246:refnum<vi>, error out=w247:errorcluster)  [unwired: 1 in, 3 out]
            n201 = property class="VI Interface Type 4"(reference=w246, error in=w247, "Front Panel Window:Open"=TRUE) -> (reference out=w251:refnum<vi>, error out=w249:errorcluster)
            n202 = call-by-ref "?"(reference=w251, error in=w249) -> (reference out=w241:refnum<vi>, error out=w240:errorcluster)  [unwired: 9 in]
            n203 = Close Reference(reference=w241, error in (no error)=w240) -> ()  [unwired: 1 out]
            n204 = event-data("Discard?"=TRUE) -> ()  [unwired: 1 in, 4 out]
          }
          event Mouse Down? {
            n205 = event-data() -> ()  [unwired: 5 out]
            n206 = global read "Constants_global.vi" "EnFlo SW Folder"() -> (w255:path)
            n207 = Build Path(base path=w255, name or relative path=path "ADAM Client/Sub VIs/User_Metadata.vi") -> (appended path=w262:path)
            n208 = Open VI Reference(type specifier VI Refnum (for type only)=refnum<vi> refnum, vi path=w262) -> (vi reference=w258:refnum<vi>, error out=w259:errorcluster)  [unwired: 1 in, 3 out]
            n209 = property class="VI Interface Type 4"(reference=w258, error in=w259, "Front Panel Window:Open"=TRUE) -> (reference out=w263:refnum<vi>, error out=w261:errorcluster)
            n210 = call-by-ref "?"(reference=w263, error in=w261) -> (reference out=w253:refnum<vi>, error out=w252:errorcluster)  [unwired: 9 in]
            n211 = Close Reference(reference=w253, error in (no error)=w252) -> ()  [unwired: 1 out]
            n212 = event-data("Discard?"=TRUE) -> ()  [unwired: 1 in, 4 out]
          }
          event Mouse Down? {
            n213 = event-data() -> ()  [unwired: 5 out]
            n214 = global read "Constants_global.vi" "EnFlo SW Folder"() -> (w269:path)
            n215 = Build Path(base path=w269, name or relative path=path "ADAM Client/Sub VIs/EnFlo_Tunnel_Setup.vi") -> (appended path=w272:path)
            n216 = Open VI Reference(type specifier VI Refnum (for type only)=refnum<vi> refnum, vi path=w272) -> (vi reference=w266:refnum<vi>, error out=w265:errorcluster)  [unwired: 1 in, 3 out]
            n217 = call-by-ref "?"(reference=w266, error in=w265) -> (reference out=w268:refnum<vi>, error out=w267:errorcluster)  [unwired: 9 in]
            n218 = Close Reference(reference=w268, error in (no error)=w267) -> ()  [unwired: 1 out]
            n219 = event-data("Discard?"=TRUE) -> ()  [unwired: 1 in, 4 out]
          }
          event Mouse Down? {
            w283 = TRUE  # Show Panel?
            n220 = event-data() -> ()  [unwired: 5 out]
            n221 = global read "Constants_global.vi" "EnFlo SW Folder"() -> (w278:path)
            n222 = Build Path(base path=w278, name or relative path=path "Anemometry/Anemometry Sub Vis/Gen Trav/Traverse_Space.vi") -> (appended path=w281:path)
            n223 = global read "Trav_pos_global.vi" "Default Traverse Setup"() -> (w273:string)
            n224 = Open VI Reference(type specifier VI Refnum (for type only)=refnum<vi> refnum, vi path=w281) -> (vi reference=w282:refnum<vi>, error out=w274:errorcluster)  [unwired: 1 in, 3 out]
            n225 = call-by-ref "?"(reference=w282, error in=w274, "Show Panel?"=w283, "Traverse Setup"=w273) -> (reference out=w276:refnum<vi>, error out=w275:errorcluster)  [unwired: 8 in, 1 out]
            n226 = Close Reference(reference=w276, error in (no error)=w275) -> ()  [unwired: 1 out]
            n227 = event-data("Discard?"=TRUE) -> ()  [unwired: 1 in, 4 out]
          }
          event Mouse Down? {
            n228 = event-data() -> ()  [unwired: 5 out]
            n229 = global read "Constants_global.vi" "EnFlo SW Folder"() -> (w285:path)
            n230 = Build Path(base path=w285, name or relative path=path "Anemometry/Anemometry Sub Vis/Traverse vi's/EnFlo Tunnel specific/Check_EnFlo_Arm.vi") -> (appended path=w287:path)
            n231 = call "Open_Close_Front_Panel.ph.vi"("Front Panel Window:Open"=TRUE, "VI path"=w287) -> ()  [unwired: 2 out]
            n232 = event-data() -> ()  [unwired: 1 in, 2 out]
          }
          event Mouse Down? {
            n233 = event-data() -> ()  [unwired: 5 out]
            n234 = global read "Constants_global.vi" "EnFlo SW Folder"() -> (w295:path)
            n235 = Build Path(base path=w295, name or relative path=path "Anemometry/Anemometry Sub Vis/Gen Trav/3D_Traverse_move.vi") -> (appended path=w292:path)
            n236 = Strip Path(path=w292) -> (name=w291:string)  [unwired: 1 out]
            n237 = Open VI Reference(vi path=w291) -> (vi reference=w293:refnum<vi>, error out=w294:errorcluster)  [unwired: 1 in, 4 out]
            n238 = property class="VI"(reference=w293, error in=w294) -> (reference out=w289:refnum<vi>, error out=w288:errorcluster, "Front Panel Window:Open"=w290:bool)
            n239 = case shown="False" w290 {
              tunnel: w292 -> [w297 _]
              tunnel: w289 -> [_ w314]
              tunnel: w288 -> [_ w313]
              frame False {
                n240 = global read "Trav_pos_global.vi" "Work in Tunnel Coordinates?"() -> (w307:T47)
                n241 = global read "Trav_pos_global.vi" "Default Traverse Setup"() -> (w305:string)
                n242 = Open VI Reference(type specifier VI Refnum (for type only)=refnum<vi> refnum, vi path=w297) -> (vi reference=w301:refnum<vi>, error out=w302:errorcluster)  [unwired: 1 in, 3 out]
                n243 = property class="VI Interface Type 5"(reference=w301, error in=w302, "Front Panel Window:Open"=TRUE) -> (reference out=w298:refnum<vi>, error out=w299:errorcluster)
                n244 = call-by-ref "?"(reference=w298, error in=w299, "Mode"=Trav_mode."Read traverse position", "Work in Tunnel Coordinates"=w307, "Simulate/Run"=User_Specific_mode."Run VI", "Traverse name"=w305) -> (reference out=w303:refnum<vi>, error out=w304:errorcluster)  [unwired: 9 in, 3 out]
                n245 = Close Reference(reference=w303, error in (no error)=w304) -> ()  [unwired: 1 out]
              }
              frame True {
                n246 = property class="VI"(reference=w314, error in=w313, "Front Panel Window:Open"=TRUE) -> (reference out=w312:refnum<vi>, error out=w311:errorcluster)
                n247 = Close Reference(reference=w312, error in (no error)=w311) -> ()  [unwired: 1 out]
              }
            }
            n248 = event-data() -> ()  [unwired: 1 in, 5 out]
          }
          event Mouse Down? {
            n249 = event-data() -> ()  [unwired: 5 out]
            n250 = Open VI Reference(vi path="Multi_Run_Prog.vi") -> (vi reference=w320:refnum<vi>, error out=w319:errorcluster)  [unwired: 1 in, 4 out]
            n251 = property class="VI"(reference=w320, error in=w319, "Front Panel Window:Open"=TRUE) -> (reference out=w317:refnum<vi>, error out=w318:errorcluster)
            n252 = Close Reference(reference=w317, error in (no error)=w318) -> (error out=w315:errorcluster)
            n253 = Unbundle By Name(w315) -> ("status"=w322:bool)
            n254 = case shown="False" w322 {
              frame False {
              }
              frame True {
                n255 = global read "Constants_global.vi" "General folder"() -> (w329:path)
                n256 = global read "Constants_global.vi" "EnFlo SW Folder"() -> (w330:path)
                n257 = Build Path(base path=w329, name or relative path="Multi_Run_Filename.txt") -> (appended path=w326:path)
                n258 = Build Path(base path=w330, name or relative path=path "Anemometry/Multi_Run_Prog.vi") -> (appended path=w327:path)
                n259 = call "Read_File_Simple.vi"("Filename"=w326) -> ("string"=w325:string)  [unwired: 2 in, 7 out]
                n260 = String To Path(string=w325) -> (path=w323:path)
                n261 = call "Does_file_exist_(simple).vi"("Pathname"=w323) -> ("exists?"=w324:bool)
                n262 = case shown="False" w324 {
                  tunnel: w327 -> [w332 w344]
                  tunnel: w323 -> [_ w341]
                  frame False {
                    n263 = call "Open_Close_Front_Panel.ph.vi"("Front Panel Window:Open"=TRUE, "VI path"=w332) -> ()  [unwired: 2 out]
                  }
                  frame True {
                    n264 = Open VI Reference(type specifier VI Refnum (for type only)=refnum<vi> refnum, vi path=w344) -> (vi reference=w340:refnum<vi>, error out=w339:errorcluster)  [unwired: 1 in, 3 out]
                    n265 = property class="VI Interface Type 6"(reference=w340, error in=w339, "Front Panel Window:Open"=TRUE) -> (reference out=w337:refnum<vi>, error out=w338:errorcluster)
                    n266 = call-by-ref "?"(reference=w337, error in=w338, "Command filename"=w341, "Setup mode"=T45."Load Command File") -> (reference out=w336:refnum<vi>, error out=w335:errorcluster)  [unwired: 18 in]
                    n267 = Close Reference(reference=w336, error in (no error)=w335) -> ()  [unwired: 1 out]
                  }
                }
              }
            }
            n268 = event-data() -> ()  [unwired: 1 in, 5 out]
          }
          event Mouse Down? {
            w346 = "Calibration.vi" ("name or relative path")
            n269 = event-data() -> ()  [unwired: 5 out]
            n270 = global read "Constants_global.vi" "EnFlo SW Folder"() -> (w352:path)
            n271 = Open VI Reference(vi path=w346) -> (vi reference=w350:refnum<vi>, error out=w349:errorcluster)  [unwired: 1 in, 4 out]
            n272 = Build Path(base path=w352, name or relative path="Anemometry") -> (appended path=w355:path)
            n273 = property class="VI"(reference=w350, error in=w349, "Front Panel Window:Open"=TRUE) -> (reference out=w347:refnum<vi>, error out=w348:errorcluster)
            n274 = Build Path(base path=w355, name or relative path=w346) -> (appended path=w353:path)
            n275 = Close Reference(reference=w347, error in (no error)=w348) -> (error out=w345:errorcluster)
            n276 = Unbundle By Name(w345) -> ("status"=w354:bool)
            n277 = case shown="True" w354 {
              tunnel: w353 -> [_ w357]
              tunnel: w345 -> [_ _]
              frame False {
              }
              frame True {
                n278 = stacked-sequence {
                  seq-local: [w361 _] -> [_ w370]
                  tunnel: w357 -> [_ w371]
                  frame #0 {
                    n279 = global read "Constants_global.vi" "Calib setups folder"() -> (w366:path)
                    n280 = Build Path(base path=w366, name or relative path="Current_Setup.xls") -> (appended path=w359:path)
                    n281 = call "Read_File_Simple.vi"("Filename"=w359) -> ("string"=w367:string)  [unwired: 2 in, 7 out]
                    n282 = Format Into String(format string="Calibration Setup File   %s", w359) -> (resulting string=w358:string)  [unwired: 2 in, 1 out]
                    n283 = call "Get_string_subset.vi"("String Name"=w358, "String to split"=w367, "File Label"="Raw data header") -> ("Output string"=w363:string)  [unwired: 1 in, 1 out]
                    n284 = call "Get_Characters_from_string.vi"("Input string"=w363, "Variable name"="Calib filename") -> ("Value"=w362:string)  [unwired: 1 in, 1 out]
                    n285 = call "String_to_Pathname.vi"("Input String"=w362) -> ("path"=w361:path)
                  }
                  frame #1 {
                    n286 = call "Does_file_exist_(simple).vi"("Pathname"=w370) -> ("exists?"=w369:bool)
                    n287 = case shown="True" w369 {
                      tunnel: w371 -> [w372 w387]
                      tunnel: w370 -> [_ w381]
                      frame False {
                        n288 = call "Open_Close_Front_Panel.ph.vi"("Front Panel Window:Open"=TRUE, "VI path"=w372) -> ()  [unwired: 2 out]
                      }
                      frame True {
                        w379 = TRUE ("Front Panel Window:Open")
                        n289 = Open VI Reference(type specifier VI Refnum (for type only)=refnum<vi> refnum, vi path=w387) -> (vi reference=w385:refnum<vi>, error out=w380:errorcluster)  [unwired: 1 in, 3 out]
                        n290 = property class="VI Interface Type 7"(reference=w385, error in=w380, "Front Panel Window:Open"=w379, "Front Panel Window:Auto Center (Deprecated)"=w379) -> (reference out=w384:refnum<vi>, error out=w383:errorcluster)
                        n291 = call-by-ref "?"(reference=w384, error in=w383, "Mode"=Calib_mode."Setup Front Panel", "Calib file"=w381) -> (reference out=w377:refnum<vi>, error out=w376:errorcluster)  [unwired: 15 in, 3 out]
                        n292 = property class="VI Interface Type 7"(reference=w377, error in=w376, "Front Panel Window:Auto Center (Deprecated)"=FALSE ("Front Panel Window:Auto Center")) -> (reference out=w375:refnum<vi>, error out=w374:errorcluster)
                        n293 = Close Reference(reference=w375, error in (no error)=w374) -> ()  [unwired: 1 out]
                      }
                    }
                  }
                }
              }
            }
            n294 = event-data() -> ()  [unwired: 1 in, 5 out]
          }
          event "stop": Mouse Down? {
            n295 = event-data() -> ()  [unwired: 5 out]
            n296 = flat-sequence {
              frame #0 {
                n297 = global write "Dynamic_call_global.ph.vi" "EnFlo Hub running?"(FALSE ("EnFlo Hub running?")) -> ()
              }
              frame #1 {
                n298 = Stop(stop? (T)=TRUE) -> ()
              }
            }
            n299 = event-data() -> ()  [unwired: 1 in, 4 out]
          }
          event "Rig_Control": Value Change {
            n300 = event-data() -> ("OldVal"=w391:cluster{"Ch Name":string, "Boolean":bool}[], "NewVal"=w390:cluster{"Ch Name":string, "Boolean":bool}[])  [unwired: 5 out]
            n301 = for {
              tunnel: w391 -> [w397] mode=indexing
              tunnel: w390 -> [w396] mode=indexing
              n302 = Unbundle By Name(w397) -> ("Ch Name"=w394:string, "Boolean"=w395:bool)
              n303 = Unbundle By Name(w396) -> ("Boolean"=w393:bool)  [unwired: 1 out]
              n304 = Not Equal?(x=w395, y=w393) -> (x != y?=w392:bool)
              n305 = case shown="True" w392 {
                tunnel: w394 -> [_ w399]
                tunnel: w393 -> [_ w406]
                frame False {
                }
                frame True {
                  n306 = Select(t="TRUE", s=w406, f="FALSE") -> (s? t:f=w398:string)
                  n307 = Select(t=1.0, s=w406, f=0.0) -> (s? t:f=w405:dbl)
                  n308 = Format Into String(format string="Are you sure you want to make %s %s?", w399, w398) -> (resulting string=w408:string)  [unwired: 2 in, 1 out]
                  n309 = Format Into String(format string="Make  %s  %s", w399, w398) -> (resulting string=w400:string)  [unwired: 2 in, 1 out]
                  n310 = Two Button Dialog(message=w408, 1:w400, 2:"Cancel" ("T button name (\"OK\")")) -> (T button?=w402:bool)
                  n311 = case shown="False" w402 {
                    tunnel: w399 -> [w413 _]
                    tunnel: w405 -> [w412 _]
                    frame False {
                      n312 = Build Array(w412) -> (w415:dbl[])
                      n313 = Build Array(w413) -> (w414:string[])
                      n314 = call "ASYNC_Adam_client.vi"("Values"=w415, "Channel Names"=w414) -> ()  [unwired: 2 out]
                    }
                    frame True {
                    }
                  }
                }
              }
            }
          }
          event Mouse Down? {
            w422 = TRUE  # Show Panel
            n315 = event-data() -> ()  [unwired: 5 out]
            n316 = global read "Constants_global.vi" "EnFlo SW Folder"() -> (w416:path)
            n317 = Build Path(base path=w416, name or relative path=path "Anemometry/Anemometry Sub Vis/LDA/Enter_LDA_Setup.vi") -> (appended path=w420:path)
            n318 = Open VI Reference(type specifier VI Refnum (for type only)=refnum<vi> refnum, vi path=w420) -> (vi reference=w423:refnum<vi>, error out=w424:errorcluster)  [unwired: 1 in, 3 out]
            n319 = call-by-ref "?"(reference=w423, error in=w424, "Show Panel"=w422) -> (reference out=w418:refnum<vi>, error out=w419:errorcluster)
            n320 = Close Reference(reference=w418, error in (no error)=w419) -> ()  [unwired: 1 out]
            n321 = event-data() -> ()  [unwired: 1 in, 4 out]
          }
        }
      }
    }
    "Numeric" <- w9
  }
  n322 = while {
    shift-left: _ -> [w430]
    shift-right: [w431] -> _
    shift-left: "Initialise" -> [w429]
    shift-right: [w432] -> _
    tunnel: "ADAM_Chs_to_Enable.txt" ("name or relative path") -> [w427]
    tunnel: "ADAM_Chs_to_View.txt" ("name or relative path") -> [w426]
    tunnel: "ResultsHierarchy.txt" ("name or relative path") -> [w425]
    i -> [w428]
    stop <- TRUE continue-if-true
    n323 = case shown="\"Initialise\"" w429 {
      tunnel: ["End" "Initialise" "Wait for call remote sub vi occurrence" "Check type of VI to launch" w510 "Wait until remote sub vi is opened" "Update opened vis array" "Update opened vis array" "Update opened vis array" "Wait until remote sub vi is opened" "Wait for call remote sub vi occurrence"] -> w432
      tunnel: [w434 w449 w455 errorcluster {"status"=FALSE, "code"=0, "source"=""} ("error out") w506 w521 w551 w568 w583 w623 w643] -> w431
      tunnel: w430 -> [w434 w449 w455 _ w506 w521 _ _ _ w623 w643]
      tunnel: w429 -> [w436 _ _ _ _ _ _ _ _ _ _]
      tunnel: w428 -> [_ _ _ _ _ _ _ _ _ _ _]
      tunnel: w427 -> [_ _ w452 _ _ _ _ _ _ _ _]
      tunnel: w426 -> [_ _ w451 _ _ _ _ _ _ _ _]
      tunnel: w425 -> [_ _ w450 _ _ _ _ _ _ _ _]
      frame "No match", Default {
        n324 = Current VI's Path() -> (path=w437:path)
        n325 = Format Into String(format string="The Case\"%s\" was not Matched\nin VI named\n'%s\"" ("Format String"), w436, w437) -> (resulting string=w440:string)  [unwired: 2 in, 1 out]
        n326 = One Button Dialog(message=w440, button name ("OK")="STOP") -> (true=w438:bool)
        n327 = Stop(stop? (T)=w438) -> ()
      }
      frame "Never run" {
        # "These globals are here to make sure they stay in momory\nafter \"Preference Panel\" has finished running"
        n328 = call "Email_With_Log.vi"() -> ()  [unwired: 4 in, 3 out]
        n329 = call "Remember_value.vi"() -> ()  [unwired: 3 in, 1 out]
        n330 = call "Read_Write_Local_table.vi"() -> ()  [unwired: 3 in, 3 out]
        n331 = call "Overhead_Factor.vi"() -> ()  [unwired: 4 in, 1 out]
        n332 = global read "Trav_pos_global.vi" "Dummy Measurement?"() -> (→"Dummy Measurement":bool)
        n333 = global read "PWAtasksGLOBAL.vi" "Analogue Dev Name"() -> (→"Analogue Dev Name":string)
        n334 = global read "Constants_global.vi" "Meas setups folder"() -> (→"Meas setups folder":path)
        n335 = global read "Dynamic_call_global.ph.vi" "Ready to take data?"() -> (→"Ready to take data?":T1)
        n336 = global read "Qnet_Globals.vi" "Local Site Root"() -> (→"Local Site Root":path)
        n337 = global read "Preference_global.vi" "Rig Setup"() -> (→"Rig Name":string)
      }
      frame "Initialise" {
        n338 = stacked-sequence {
          tunnel: w452 -> [_ _ _ _ w498]
          tunnel: w451 -> [_ _ _ _ w495]
          tunnel: w450 -> [_ _ _ _ w491]
          frame #0 {
            n339 = Generate Occurrence() -> (w477:refnum<k4>)
            n340 = global write "Dynamic_call_global.ph.vi" "Call Remote Subvi"(w477) -> ()
            n341 = Generate Occurrence() -> (w476:refnum<k4>)
            n342 = global write "Dynamic_call_global.ph.vi" "Remote Subvi Opened"(w476) -> ()
            n343 = Initialize Array("", 0) -> (w474:string[])
            n344 = global write "Dynamic_call_global.ph.vi" "Opened VIs"(w474) -> ()
            n345 = global write "Email_transfer_global.vi" "Busy?"(FALSE ("Busy?")) -> ()
            n346 = Current VI's Path() -> (path=w466:path)
            n347 = Strip Path(path=w466) -> (stripped path=w464:path)  [unwired: 1 out]
            n348 = Build Path(base path=w464, name or relative path="Utilities") -> (appended path=w462:path)
            n349 = Build Path(base path=w462, name or relative path="Preference_Panel.vi") -> (appended path=w461:path)
            n350 = Get Date/Time In Seconds() -> (seconds since 1Jan1904=w472:timestamp)
            n351 = To Double Precision Float(number=w472) -> (double precision float=w471:dbl)
            n352 = Open VI Reference(type specifier VI Refnum (for type only)=refnum<vi> refnum, vi path=w461) -> (vi reference=w467:refnum<vi>, error out=w468:errorcluster)  [unwired: 1 in, 3 out]
            n353 = Generate Occurrence() -> (w457:refnum<k4>)
            n354 = global write "Meas_global.vi" "Start Time of experiment"(w471) -> ()
            n355 = global write "Meas_global.vi" "Post Process"(Post_Process."Post Process Raw Data File" ("Post Process")) -> ()
            n356 = call-by-ref "?"(reference=w467, error in=w468, "Mode"=Preference_Mode."Load Preferences from file") -> (reference out=w469:refnum<vi>, error out=w470:errorcluster)
            n357 = global write "Dynamic_call_global.ph.vi" "Take data"(w457) -> ()
            n358 = Close Reference(reference=w469, error in (no error)=w470) -> ()  [unwired: 1 out]
          }
          frame #1 {
            w478 = TRUE  # OK
            n359 = call "Get_users_email_addresses.vi"("OK"=w478) -> ()  [unwired: 5 out]
          }
          frame #2 {
            n360 = Current VI's Path() -> (path=w487:path)
            n361 = Open VI Reference(vi path=w487) -> (vi reference=w486:refnum<vi>, error out=w485:errorcluster)  [unwired: 1 in, 4 out]
            n362 = call "Last_modified_date.vi"("Update Now"=TRUE) -> ("Programs last revision time"=w480:u32)  [unwired: 1 out]
            n363 = property class="VI"(reference=w486, error in=w485, "Front Panel Window:Open"=TRUE, "Front Panel Window:Is Frontmost"=FALSE) -> (reference out=w484:refnum<vi>, error out=w483:errorcluster)
            n364 = global write "Meas_global.vi" "Prog's last revision date"(w480) -> ()
            n365 = Close Reference(reference=w484, error in (no error)=w483) -> ()  [unwired: 1 out]
          }
          frame #3 {
            n366 = global write "Dynamic_call_global.ph.vi" "EnFlo Hub running?"(TRUE ("EnFlo Hub running?")) -> ()
          }
          frame #4 {
            # "If file not found, default values could be sent to global:"
            # "Contents of Surrey ResultsHierarchy.txt:"
            # "Year;Rig;User;DataType;Month-Year"
            n367 = global read "Constants_global.vi" "All_Users"() -> (w492:path)
            n368 = Build Path(base path=w492, name or relative path=w495) -> (appended path=w497:path)
            n369 = Build Path(base path=w492, name or relative path=w491) -> (appended path=w490:path)
            n370 = Build Path(base path=w492, name or relative path=w498) -> (appended path=w500:path)
            n371 = call "Read_File_Simple.vi"("Filename"=w497) -> ("string"=w496:string)  [unwired: 2 in, 7 out]
            n372 = call "Read_File_Simple.vi"("Filename"=w490) -> ("string"=w493:string)  [unwired: 2 in, 7 out]
            n373 = call "Read_File_Simple.vi"("Filename"=w500) -> ("string"=w501:string)  [unwired: 2 in, 7 out]
            n374 = call "Get_array_values_fr_String.vi"("String Value"=w496) -> ("String array"=→"List of ADAM channels to view":string[])  [unwired: 1 out]
            n375 = call "Get_array_values_fr_String.vi"("String Value"=w493) -> ("String array"=w489:string[])  [unwired: 1 out]
            n376 = call "Get_array_values_fr_String.vi"("String Value"=w501) -> ("String array"=→"List of ADAM control channels":string[])  [unwired: 1 out]
            n377 = global write "Preference_global.vi" "ResultsHierarchy"(w489) -> ()
          }
        }
        "Iterations" <- 0 ("Iterations")
      }
      frame "Wait for call remote sub vi occurrence" {
        n378 = global read "Dynamic_call_global.ph.vi" "Call Remote Subvi"() -> (w504:refnum<k4>)
        n379 = Wait on Occurrence(2:w504) -> ()  [unwired: 3 out]
      }
      frame "Check type of VI to launch" {
        n380 = global read "Dynamic_call_global.ph.vi" "VI name to launch"() -> (w508:string)
        n381 = Match Pattern(string=w508, regular expression=";") -> (before substring=w505:string, after substring=w507:string)  [unwired: 3 out]
        n382 = case shown="\"Open LDA PWA & An\"" w505 {
          tunnel: ["Open vi" "Open application reference" "Open Analogue input server" w518] -> w510
          tunnel: [w513 w515 w517 w519] -> w509
          tunnel: w508 -> [w513 _ _ _]
          tunnel: w507 -> [_ w515 w517 w519]
          tunnel: w505 -> [_ _ _ w518]
          frame "Other", Default {
          }
          frame "Open Application Reference" {
          }
          frame "Open Analogue Input VI" {
          }
          frame "Open LDA PWA & An" {
          }
        }
        "VI Name" <- w509
      }
      frame "Open application reference" {
        n383 = local read "VI Name"() -> (w522:string)
        n384 = Match Pattern(string=w522, regular expression=";") -> (before substring=w530:string, after substring=w531:string)  [unwired: 3 out]
        n385 = Decimal String To Number(string=w531) -> (number=w532:i32)  [unwired: 3 out]
        n386 = To Unsigned Long Integer(number=w532) -> (unsigned 32bit integer=w529:u32)
        n387 = call "App_Ref_Global.vi"("Mode"=App_Global."Read Global") -> ("Output Array"=w528:T49[])  [unwired: 1 in, 1 out]
        n388 = Open Application Reference(10:w529, 11:w530) -> (0:w523:errorcluster, 3:w527:refnum<vi>)  [unwired: 1 in, 1 out]
        n389 = for {
          tunnel: w528 -> [w534] mode=indexing
          tunnel: w522 -> [w538]
          tunnel: w527 -> [w536]
          tunnel: [w535] -> w526 mode=indexing
          n390 = Unbundle By Name(w534) -> ("Server IP & Port No"=w539:string)
          n391 = Equal?(x=w539, y=w538) -> (x = y?=w537:bool)
          n392 = case shown="False" w537 {
            tunnel: w536 -> [_ w543]
            tunnel: [w540 w542] -> w535
            tunnel: w534 -> [w540 w541]
            frame False {
            }
            frame True {
              n393 = Bundle By Name(cluster=w541, "Application reference"=w543) -> (w542:T49)
            }
          }
        }
        n394 = global write "Dynamic_call_global.ph.vi" "Error Cluster"(w523) -> ()
        n395 = call "App_Ref_Global.vi"("Input Array"=w526, "Mode"=App_Global."Write to Global") -> ()  [unwired: 2 out]
      }
      frame "Open Analogue input server" {
        n396 = local read "VI Name"() -> (w548:string)
        n397 = call "Get_link_info.vi"("VI Name"=w548) -> ("Path name"=w545:path, "Application reference"=w546:refnum<vi>, "Local Call?"=w547:bool)  [unwired: 1 out]
        n398 = global read "Dynamic_call_global.ph.vi" "Analogue Input"() -> (w550:refnum<vi>)
        n399 = case shown="True" w547 {
          tunnel: w550 -> [w556 w560]
          tunnel: [w552 w559] -> w549
          tunnel: [w555 w558] -> w551
          tunnel: w548 -> [w554 _]
          tunnel: w546 -> [w553 _]
          tunnel: w545 -> [_ w557]
          frame False {
            n400 = Open VI Reference(type specifier VI Refnum (for type only)=w556, application reference (local)=w553, vi path=w554) -> (vi reference=w552:refnum<vi>, error out=w555:errorcluster)  [unwired: 1 in, 2 out]
          }
          frame True {
            n401 = Open VI Reference(type specifier VI Refnum (for type only)=w560, vi path=w557) -> (vi reference=w559:refnum<vi>, error out=w558:errorcluster)  [unwired: 1 in, 3 out]
          }
        }
        n402 = global write "Dynamic_call_global.ph.vi" "Analogue Input"(w549) -> ()
      }
      frame "Open LDA PWA & An" {
        n403 = local read "VI Name"() -> (w565:string)
        n404 = call "Get_link_info.vi"("VI Name"=w565) -> ("Path name"=w562:path, "Application reference"=w563:refnum<vi>, "Local Call?"=w564:bool)  [unwired: 1 out]
        n405 = global read "Dynamic_call_global.ph.vi" "Take LDA PWA & An"() -> (w567:refnum<vi>)
        n406 = case shown="True" w564 {
          tunnel: w567 -> [w573 w577]
          tunnel: [w569 w576] -> w566
          tunnel: [w572 w575] -> w568
          tunnel: w565 -> [w571 _]
          tunnel: w563 -> [w570 _]
          tunnel: w562 -> [_ w574]
          frame False {
            n407 = Open VI Reference(type specifier VI Refnum (for type only)=w573, application reference (local)=w570, vi path=w571) -> (vi reference=w569:refnum<vi>, error out=w572:errorcluster)  [unwired: 1 in, 2 out]
          }
          frame True {
            n408 = Open VI Reference(type specifier VI Refnum (for type only)=w577, vi path=w574) -> (vi reference=w576:refnum<vi>, error out=w575:errorcluster)  [unwired: 1 in, 3 out]
          }
        }
        n409 = global write "Dynamic_call_global.ph.vi" "Take LDA PWA & An"(w566) -> ()
      }
      frame "Open vi" {
        n410 = local read "VI Name"() -> (w582:string)
        n411 = call "Get_link_info.vi"("VI Name"=w582) -> ("Path name"=w581:path, "Application reference"=w580:refnum<vi>, "Local Call?"=w579:bool)  [unwired: 1 out]
        n412 = case shown="\"No Match\", Default" w582 {
          tunnel: [w584 w593 w605] -> w583
          tunnel: w582 -> [w589 w592 w609]
          tunnel: w581 -> [_ _ w606]
          tunnel: w580 -> [_ w591 w608]
          tunnel: w579 -> [_ w590 w607]
          frame "No Match", Default {
            n413 = Format Into String(format string="VI named \"%s\" Not matched" ("Format String"), w589) -> (resulting string=w586:string)  [unwired: 2 in, 1 out]
            n414 = Bundle By Name(cluster=errorcluster {"status"=FALSE, "code"=0, "source"=""} ("error out"), "source"=w586, "status"=TRUE ("Bundle Element")) -> (w584:errorcluster)
          }
          frame "Program_Active_server.vi" {
            n415 = global read "Dynamic_call_global.ph.vi" "Program Active server"() -> (w595:refnum<vi>)
            n416 = case shown="True" w590 {
              tunnel: w595 -> [w600 w604]
              tunnel: [w599 w603] -> w594
              tunnel: [w598 w602] -> w593
              tunnel: w592 -> [w597 w601]
              tunnel: w591 -> [w596 _]
              frame False {
                n417 = Open VI Reference(type specifier VI Refnum (for type only)=w600, application reference (local)=w596, vi path=w597) -> (vi reference=w599:refnum<vi>, error out=w598:errorcluster)  [unwired: 1 in, 2 out]
              }
              frame True {
                n418 = Open VI Reference(type specifier VI Refnum (for type only)=w604, vi path=w601) -> (vi reference=w603:refnum<vi>, error out=w602:errorcluster)  [unwired: 1 in, 3 out]
              }
            }
            n419 = global write "Dynamic_call_global.ph.vi" "Program Active server"(w594) -> ()
          }
          frame "GPIB_Server.vi" {
            n420 = global read "Dynamic_call_global.ph.vi" "GPIB_Server.vi"() -> (w611:refnum<vi>)
            n421 = case shown="False" w607 {
              tunnel: w611 -> [w616 w620]
              tunnel: [w615 w619] -> w610
              tunnel: [w614 w618] -> w605
              tunnel: w609 -> [w612 _]
              tunnel: w608 -> [w613 _]
              tunnel: w606 -> [_ w617]
              frame False {
                n422 = Open VI Reference(type specifier VI Refnum (for type only)=w616, application reference (local)=w613, vi path=w612) -> (vi reference=w615:refnum<vi>, error out=w614:errorcluster)  [unwired: 1 in, 2 out]
              }
              frame True {
                n423 = Open VI Reference(type specifier VI Refnum (for type only)=w620, vi path=w617) -> (vi reference=w619:refnum<vi>, error out=w618:errorcluster)  [unwired: 1 in, 3 out]
              }
            }
            n424 = global write "Dynamic_call_global.ph.vi" "GPIB_Server.vi"(w610) -> ()
          }
        }
      }
      frame "Update opened vis array" {
        w625 = TRUE  # Dialog Box
        n425 = local read "VI Name"() -> (w624:string)
        n426 = Unbundle By Name(w623) -> ("status"=w628:bool, "source"=w626:string)
        n427 = case shown="True" w628 {
          tunnel: w623 -> [w630 w639]
          tunnel: [w630 w638] -> w627
          tunnel: w624 -> [w631 w634]
          tunnel: w626 -> [_ w637]
          frame False {
            n428 = global read "Dynamic_call_global.ph.vi" "Opened VIs"() -> (w632:string[])
            n429 = To Upper Case(1:w631) -> (0:w629:string)
            n430 = Build Array (concatenate)(w632, w629) -> (w633:string[])
            n431 = global write "Dynamic_call_global.ph.vi" "Opened VIs"(w633) -> ()
          }
          frame True {
            n432 = Concatenate Strings(w634, " " ("Substring"), w637) -> (w635:string)
            n433 = Bundle By Name(cluster=w639, "source"=w635) -> (w638:errorcluster)
          }
        }
        n434 = call "EnFlo_Error_Handler.vi"("error in (no error)"=w627, "Error Type"="Dynamic Call", "Dialog Box (T)"=w625) -> ()  [unwired: 3 out]
      }
      frame "Wait until remote sub vi is opened" {
        n435 = global read "Dynamic_call_global.ph.vi" "Remote Subvi Opened"() -> (w644:refnum<k4>)
        n436 = local read "Iterations"() -> (w642:i32)
        n437 = Increment(x=w642) -> (x+1=w641:i32)
        n438 = local write "Iterations"(w641) -> ()
        n439 = Set Occurrence(w644) -> ()
      }
    }
  }
  n440 = while {
    stop <- FALSE stop-if-true
    n441 = global read "Dynamic_call_global.ph.vi" "EnFlo Hub running?"() -> (w646:bool)
    n442 = Equal?(x="Tab Control", y=T2."Adam Table" ("Tab Control")) -> (x = y?=w647:bool)
    n443 = And(x=w647, y=w646) -> (x .and. y?=w645:bool)
    n444 = case shown="True" w645 {
      frame True {
        n445 = local read "List of ADAM channels to view"() -> (w658:string[])
        n446 = local read "List of ADAM control channels"() -> (w661:string[])
        n447 = Build Array (concatenate)(w661, w658) -> (w660:string[])
        n448 = call "Get_Current_Scan_client.vi"("ADAM Ch Names"=w660) -> ("Ch Description Array"=w655:T50[], "Numerical Values"=w659:dbl[])  [unwired: 2 out]
        n449 = Array Size(array=w661) -> (size(s)=w656:i32)
        n450 = Array Subset(array=w655, index=w656) -> (w654:T50[])  [unwired: 1 in]
        n451 = Array Subset(array=w659, index=w656) -> (w653:dbl[])  [unwired: 1 in]
        n452 = for {
          tunnel: w654 -> [w668] mode=indexing
          tunnel: [w667] -> w652 mode=indexing
          tunnel: cluster{"Ch Name":string, "Numeric":dbl} {"Ch Name"="", "Numeric"=0.0} ("Cluster") -> [w666]
          tunnel: w653 -> [w664] mode=indexing
          n453 = Unbundle By Name(w668) -> ("Ch Name"=w665:string)
          n454 = Bundle By Name(cluster=w666, "Ch Name"=w665, "Numeric"=w664) -> (w667:cluster{"Ch Name":string, "Numeric":dbl})
        }
        "Current Values" <- w652
        n455 = for {
          N: w656 -> [_]
          tunnel: cluster{"Ch Name":string, "Boolean":bool} {"Ch Name"="", "Boolean"=FALSE} ("Cluster") -> [w675]
          tunnel: w655 -> [w674] mode=indexing
          tunnel: w659 -> [w672] mode=indexing
          tunnel: [w669] -> w662 mode=indexing
          n456 = Unbundle By Name(w674) -> ("Ch Name"=w673:string)
          n457 = Greater?(x=w672, y=0.5) -> (0:w670:bool)
          n458 = Bundle By Name(cluster=w675, "Ch Name"=w673, "Boolean"=w670) -> (w669:cluster{"Ch Name":string, "Boolean":bool})
        }
        n459 = local write "Rig_Control"(w662) -> ()
      }
      frame False {
      }
    }
    n460 = Wait (ms)(milliseconds to wait=u32 1000) -> ()  [unwired: 1 out]
  }
